vi "Load Modules.vi"(8 "error in (no error)":errorcluster) -> (0 "error out":errorcluster)   [LabVIEW 2017, in "WebServiceImporter.lvlib" / "Main Panel.lvlib"]
uses:
  <vilib>/Platform/WebService/Main Panel/Main Panel.lvlib
  <vilib>/Platform/WebService/Error Handling/Error/Operation.ctl
  <vilib>/Platform/WebService/Main Panel/Pages/Input Info/Input Info.lvlib
  <vilib>/Platform/WebService/Main Panel/Pages/Select Methods/Select Methods.lvlib
  <vilib>/Platform/WebService/Main Panel/Pages/Preview/Preview.lvlib
  <vilib>/Platform/WebService/Main Panel/Pages/Progress/Progress.lvlib
  <vilib>/Platform/WebService/Main Panel/Configuration/Configuration.lvlib
  <vilib>/Platform/WebService/Error Handling/Error Handling.lvlib
  <vilib>/Platform/WebService/Main Panel/Pages/Finish/Finish.lvlib
  <vilib>/Platform/WebService/Main Panel/Pages/Input WSDL/Input WSDL.lvlib
  <vilib>/Platform/WebService/Main Panel/Pages/Authentication/Authentication.lvlib
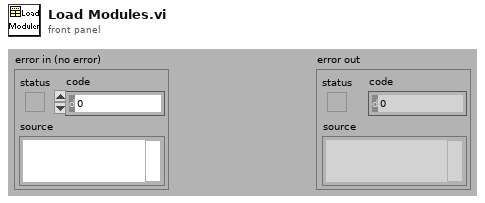
[diagram p1: front panel]
types:
  T1 = typedef "WebServiceImporter.lvlib/Error Handling.lvlib/Operation.ctl" = enum16{"Get", "Add", "Clear"}
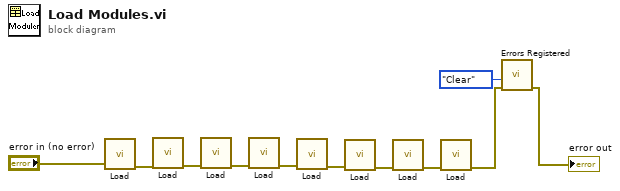
[diagram p0: block diagram]
diagram:
  n1 = call <vilib>:"Load.vi"("error in (no error)"="error in (no error)") -> ("error out"=w3:errorcluster)  [unwired: 10 in]
  n2 = call <vilib>:"Load.vi"("error in (no error)"=w3) -> ("error out"=w2:errorcluster)  [unwired: 10 in]
  n3 = call <vilib>:"Load.vi"("error in (no error)"=w2) -> ("error out"=w1:errorcluster)  [unwired: 10 in]
  n4 = call <vilib>:"Load.vi"("error in (no error)"=w1) -> ("error out"=w11:errorcluster)  [unwired: 10 in]
  n5 = call <vilib>:"Load.vi"("error in (no error)"=w11) -> ("error out"=w10:errorcluster)  [unwired: 10 in]
  n6 = call <vilib>:"Load.vi"("error in (no error)"=w10) -> ("error out"=w9:errorcluster)  [unwired: 10 in]
  n7 = call <vilib>:"Load.vi"("error in (no error)"=w9) -> ("error out"=w5:errorcluster)  [unwired: 10 in]
  n8 = call <vilib>:"Load.vi"("error in (no error)"=w5) -> ("error out"=w4:errorcluster)  [unwired: 10 in]
  n9 = call <vilib>:"Errors Registered.vi"("error in (no error)"=w4, "Operation"=Operation."Clear") -> ("error out"=→"error out":errorcluster)  [unwired: 8 in, 1 out]
